vi "PNA_RF_SRC_STATE.vi"(0 "Session In":refnum<visa-resource-name>="TCPIP0::K-Instr0000.local::hislip0::INSTR", 5 "error in":errorcluster {"code" format="%.0x"}, 7 "POW_ON(T)":bool, 8 "Timeout":u32=5000, 10 "RO(T)":bool, 11 "CH":i32=3, 13 "Source":i32=1) -> (14 "Session Out":refnum<visa-resource-name>="TCPIP0::K-Instr0000.local::hislip0::INSTR", 19 "error out":errorcluster {"code" format="%.0x"})   [LabVIEW 2018]
doc: "Applicable Models: All\n\n(Read-Write) Sets the RF power output level.\n \nParameters\n \n \n<cnum>\n Any existing channel number. If unspecified, value is set to 1\n \n<port>\n Source port number of the VNA. If unspecified, value is set to 1. To make settings for ports that are not simple numbers, use the [src] argument.\n \n<num>\n Source power in dBm.\n\nNote: The range of settable power values depends on the VNA model and if source attenuators are installed. To determine the range of values, perform a query using MAX, then MIN, as an argument. (SOUR:POW:ATT:AUTO must be set to ON) Example: SOURce:POWer? Max\n\nActual achievable leveled power depends on frequency.\n \n[src]\n String. (NOT case sensitive). Source port. Optional. Use SOUR:CAT? to return a list of valid port names.\n\nWhile this argument can be used to make settings for ALL ports, it is designed to access ports such as an external source, true mode balanced port, or one of the Source 2 outputs on the 2-port 2-source PNA-X model such as \"Port 1 Src2\". Otherwise, the <port> argument performs the same function. If both arguments are specified, [src] takes priority"
panel:
  out "mode":string
  out "concatenated string":string="sour3:pow1?\nsour3:pow1:LEV:IMM:AMPL -40.000000\n"
  # "Instrument Address"
  # "Select Source"
  # "Conditions"
  # "Is Read Only (T)"
  # "Channel"
  # "Source"
  # "Inst Timeout(ms)"
  # "Set State"
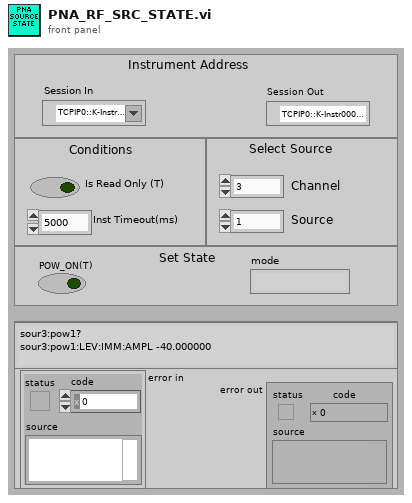
[diagram p1: front panel]
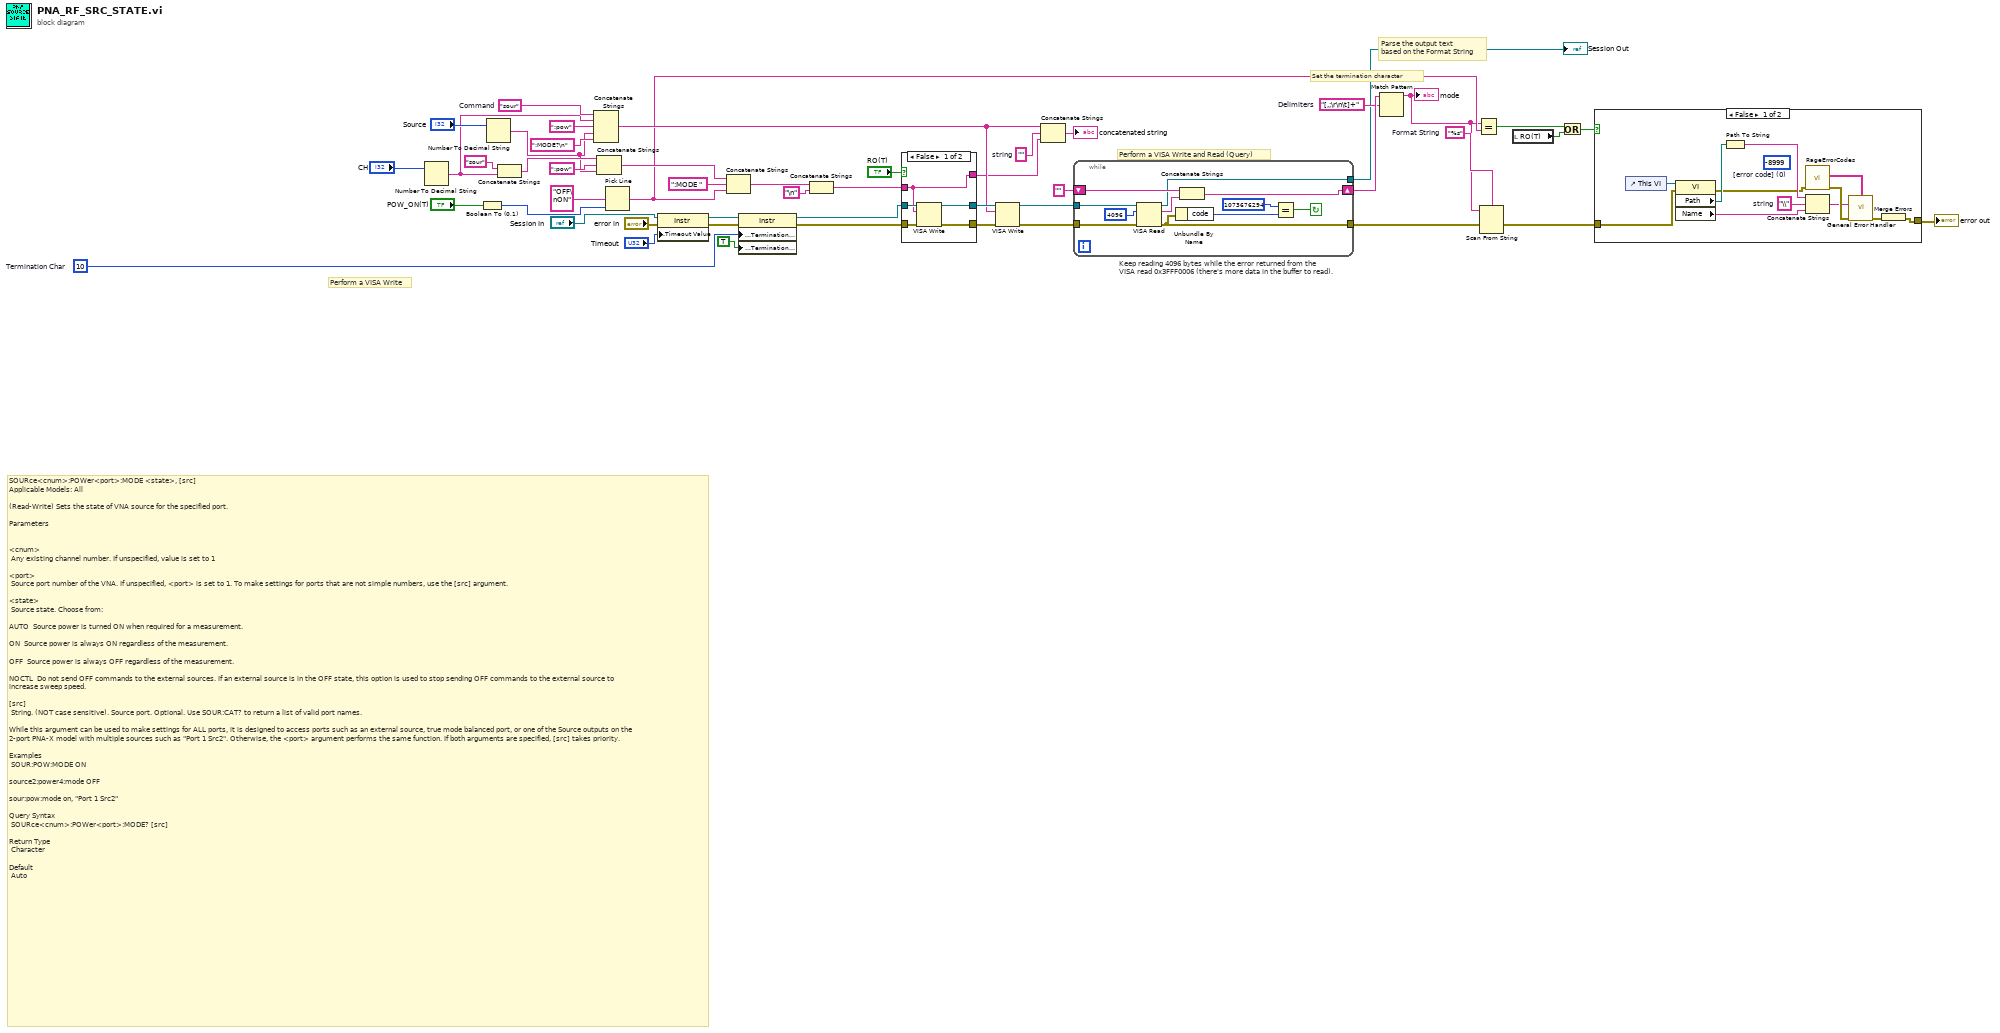
[diagram p0: block diagram]
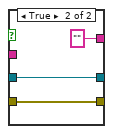
[diagram p3: hidden frame]
diagram:
  w13 = ""  # string
  w26 = "[,;\r\n\t]+"  # Delimiters
  w27 = "%s"  # Format String
  w24 = "sour"  # Command
  w43 = u8 10  # Termination Char
  # "SOURce<cnum>:POWer<port>:MODE <state>, [src]\nApplicable Models: All\n\n(Read-Write) Sets the state of VNA source for the specified port.\n \nParameters\n  \n \n<cnum>\n Any existing channel number. If unspecified, value is set to 1\n \n<port>\n Source port number of the VNA. If unspecified, <port> is set to 1. To make settings for ports that are not simple numbers, use the [src] argument.\n \n<state>\n Source state. Choose from:\n\nAUTO  Source power is turned ON when required for a measurement.\n\nON  Source power is always ON regardless of the measurement.\n\nOFF  Source power is always OFF regardless of the measurement.\n\nNOCTL  Do not send OFF commands to the external sources. If an external source is in the OFF state, this option is used to stop sending OFF commands to the external source to increase sweep speed.\n \n[src]\n String. (NOT case sensitive). Source port. Optional. Use SOUR:CAT? to return a list of valid port names.\n\nWhile this argument can be used to make settings for ALL ports, it is designed to access ports such as an external source, true mode balanced port, or one of the Source outputs on the 2-port PNA-X model with multiple sources such as \"Port 1 Src2\". Otherwise, the <port> argument performs the same function. If both arguments are specified, [src] takes priority.\n \nExamples\n SOUR:POW:MODE ON\n\nsource2:power4:mode OFF\n\nsour:pow:mode on, \"Port 1 Src2\"\n \nQuery Syntax\n SOURce<cnum>:POWer<port>:MODE? [src]\n \nReturn Type\n Character\n \nDefault\n Auto"
  # "Parse the output text based on the Format String"
  # "Perform a VISA Write and Read (Query)"
  # "Keep reading 4096 bytes while the error returned from the\nVISA read 0x3FFF0006 (there's more data in the buffer to read)."
  # "Perform a VISA Write"
  # "Set the termination character"
  n1 = Number To Decimal String(number="CH") -> (decimal integer string=w22:string)  [unwired: 1 out]
  n2 = Boolean To (0,1)(Boolean="POW_ON(T)") -> (0, 1=w4:i16)
  n3 = Number To Decimal String(number="Source") -> (decimal integer string=w17:string)  [unwired: 1 out]
  n4 = Concatenate Strings("sour" ("staticText"), w22) -> (w39:string)
  n5 = Concatenate Strings(w24, w22, ":pow" ("Command"), w17, ":MODE?\n" ("Command")) -> (w14:string)
  n6 = Concatenate Strings(w39, ":pow" ("staticText"), w17) -> (w16:string)
  n7 = Pick Line(multi-line string="OFF\nON", line index=w4) -> (output string=w2:string)  [unwired: 1 in]
  n8 = property class="Instr"(reference="Session In", error in="error in", "General Settings:Timeout Value"="Timeout") -> (reference out=w42:refnum<visa-resource-name>, error out=w45:errorcluster)
  n9 = Concatenate Strings(w16, ":MODE " ("staticText"), w2) -> (w34:string)
  n10 = property class="Instr"(reference=w42, error in=w45, "Message Based Settings:Termination Character"=w43, "Message Based Settings:Termination Character Enable"=TRUE ("enable")) -> (reference out=w25:refnum<visa-resource-name>, error out=w44:errorcluster)
  n11 = Concatenate Strings(w34, "\n" ("StaticText")) -> (w35:string)
  n12 = case shown="False" "RO(T)" {
    tunnel: w44 -> [w54 w56]
    tunnel: [w53 w56] -> w36
    tunnel: w35 -> [w50 _]
    tunnel: w25 -> [w52 w57]
    tunnel: [w51 w57] -> w21
    tunnel: [w50 ""] -> w12
    frame False {
      n13 = VISA Write(VISA resource name=w52, write buffer=w50, error in (no error)=w54) -> (VISA resource name out=w51:refnum<visa-resource-name>, error out=w53:errorcluster)  [unwired: 1 out]
    }
    frame True {
    }
  }
  n14 = VISA Write(VISA resource name=w21, write buffer=w14, error in (no error)=w36) -> (VISA resource name out=w32:refnum<visa-resource-name>, error out=w31:errorcluster)  [unwired: 1 out]
  n15 = Concatenate Strings(w14, w13, w12) -> (→"concatenated string":string)
  n16 = while {
    tunnel: w32 -> [w65]
    shift-right: [w59] -> w28
    shift-left: "" -> [w64]
    tunnel: w31 -> [w62]
    tunnel: [w61] -> w30
    tunnel: [w58] -> w20
    stop <- w60 continue-if-true
    n17 = VISA Read(VISA resource name=w65, byte count=u32 4096 ("byte count (0)"), error in (no error)=w62) -> (VISA resource name out=w58:refnum<visa-resource-name>, read buffer=w63:string, error out=w61:errorcluster)  [unwired: 1 out]
    n18 = Unbundle By Name(w61) -> ("code"=w67:i32)
    n19 = Concatenate Strings(w64, w63) -> (w59:string)
    n20 = Equal?(x=1073676294, y=w67) -> (x = y?=w60:bool)
  }
  "Session Out" <- w20
  n21 = Match Pattern(string=w28, regular expression=w26) -> (before substring=w1:string)  [unwired: 1 in, 3 out]
  "mode" <- w1
  n22 = Equal?(x=w1, y=w2) -> (x = y?=w8:bool)
  n23 = Scan From String(format string=w27, input string=w1, error in=w30) -> (error out=w10:errorcluster)  [unwired: 3 in, 2 out]
  n24 = local read "RO(T)"() -> (w7:bool)
  n25 = Or(x=w8, y=w7) -> (x .or. y?=w6:bool)
  n26 = case shown="False" w6 {
    tunnel: w10 -> [w70 w81]
    tunnel: [w71 w81] -> w9
    frame False {
      w73 = "\\"  # string
      (unwired) -8999  # [error code] (0)
      n27 = control-ref of="This VI"() -> (w78:refnum<vi>)
      n28 = property class="VI"(reference=w78, error in=w70) -> (error out=w69:errorcluster, "Path"=w76:path, "Name"=w74:string)  [unwired: 1 out]
      n29 = Path To String(path=w76) -> (string=w75:string)
      n30 = call "RageErrorCodes.vi"("error in"=w69) -> ("error out"=w80:errorcluster, "desc ary"=w79:string[])  [unwired: 8 in, 1 out]
      n31 = Concatenate Strings(w75, w73, w74) -> (w77:string)
      n32 = call <vilib>:"General Error Handler.vi"("[user-defined descriptions]"=w79, "[error source] (\" \")"=w77, "error in (no error)"=w80) -> ("error out"=w72:errorcluster)  [unwired: 8 in, 4 out]
      n33 = Merge Errors(w72) -> (w71:errorcluster)
    }
    frame True {
    }
  }
  "error out" <- w9
